vi "Load Configuration.vi"(8 "error in (no error)":errorcluster, 11 "Application in":refnum<class "Application.lvclass">) -> (0 "error out":errorcluster, 3 "Application out":refnum<class "Application.lvclass">)   [LabVIEW 2023, in "Application.lvlib" / "Application.lvclass"]
uses:
  Application.lvclass
  Application.lvclass/Application.ctl
  User Interface/Splash Screen Messages/Update Status Msg/Update Status Msg.lvclass/Update Status Msg.ctl
  <vilib>/ActorFramework/Message Enqueuer/Message Enqueuer.lvclass/Message Enqueuer.ctl
  33bbd52a-dc54-4860-8ff1-e4a75f980f2e.vi
  <vilib>/ActorFramework/Message Enqueuer/Enqueue.vi
  User Interface/Splash Screen Messages/Update Status Msg/Update Status Msg.lvclass
  C:/Program Files/National Instruments/LabVIEW 2023/vi.lib/ActorFramework/Message/Message.lvclass
  <vilib>/ActorFramework/Message Priority Queue/Priority Enqueue.vi
  Resources/GLOBAL/GLOBAL Experiment Metadata.vi
  <vilib>/Utility/xml.llb/Read From XML File(string).vi
  <vilib>/JDP Science/JSONtext/JSON text to Variant.vi
  <vilib>/JDP Science/JSONtext/LVClass Serializer/JSONtext LVClass Serializer.lvclass
panel:
  in  "Edit Button":bool
  in  "Exit":bool
  in  "OK Button":bool
  in  "Select Configuration":u16(ring) items=["Workstation"]
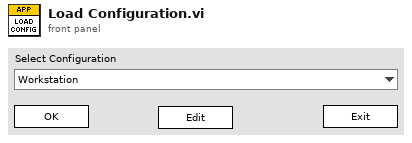
[diagram p1: front panel]
types:
  T1 = cluster{"Hostname":string[], "Config File":string[]}
  T2 = cluster{"filename without extension":string, i32}[]
  T3 = typedef "Hardware Configuration.ctl" = cluster{"Stage Configuration":T4, "Microscope Configuration":T5, "Virtual Camera Configuration":T7, "Laser Configuration":T9[], "Installed Cameras":T10[], "Power Meter Configuration":cluster{"Power Meter Type":enum16{"Disabled", "Thorlabs", "Newport", "Coherent"}, "attenuation":dbl, "instrument handle":refnum<visa-resource-name>}, "DAQ Configuration":T11}
  T4 = typedef "Stage Configuration.ctl" = cluster{"Serial Port":refnum<visa-resource-name>, "Forward Step (mm)":dbl, "Lane Length (mm)":dbl, "Lane Separation (mm)":dbl, "Stage Type":enum16{"Disabled", "ESP301", "Ti2", "Ludl", "ASI", "Simulate"}, "Autofocus Z Planes":i32, "Autofocus Range (um)":dbl, "Stage Limits":cluster{"Y Min":dbl, "Y Max":dbl, "X Min":dbl, "X Max":dbl}, "Slide (mm)":cluster{"top":dbl, "right":dbl, "width":dbl, "height":dbl}}
  T5 = typedef "Microscope Configuration.ctl" = cluster{"Serial Port":refnum<visa-resource-name>, "Microscope Type":T6, "Detection Settings":cluster{"Name":string, "Filter Position":u16, "Optical Path":u16}[]}
  T6 = typedef "Microscope Type.ctl" = enum16{"Disable", "TE2000", "Eclipse Ti", "Ti2"}
  T7 = typedef "Virtual Camera Configuration.ctl" = cluster{"Camera Type":T8}
  T8 = typedef "Camera Type.ctl" = enum16{"Hamamatsu", "Andor", "Photometrics"}
  T9 = typedef "Laser Configuration.ctl" = cluster{"Serial Port":refnum<visa-resource-name>, "Laser Type":enum16{"Disable", "Laser Quantum", "Coherent OBIS", "PRM1-Z8", "Coherent HOPS", "Cobolt"}, "Polarizer Amplitude":dbl, "Polarizer Theta Zero":dbl, "Wavelength":u16}
  T10 = typedef "Physical Camera Assignment.ctl" = cluster{"Channel Name":string, "Serial Number":string, "Flip Vertically":bool, "Flip Horizontally":bool, "wavelength":i16, "photonsPerCount":dbl[]}
  T11 = typedef "DAQ Configuration.ctl" = cluster{"Shutters":T12[], "fluidics trigger line":tag, "camera trigger line":tag, "COM Port":refnum<visa-resource-name>, "Device type":T13}
  T12 = typedef "Shutter Configuration.ctl" = cluster{"IO Line":tag, "Name":string, "Wavelength":u16, "Max rate (Hz)":dbl}
  T13 = typedef "Sync Device Type.ctl" = enum16{"Disabled", "NI DAQ", "Arduino DAQ", "Microsync"}
  T14 = typedef "Default Settings.ctl" = cluster{"Refresh Timeout (ms)":i32, "Version String":string, "Hardware Configuration File":string, "Config Hostname Map":cluster{"Hostname":string[], "Config File":string[]}}
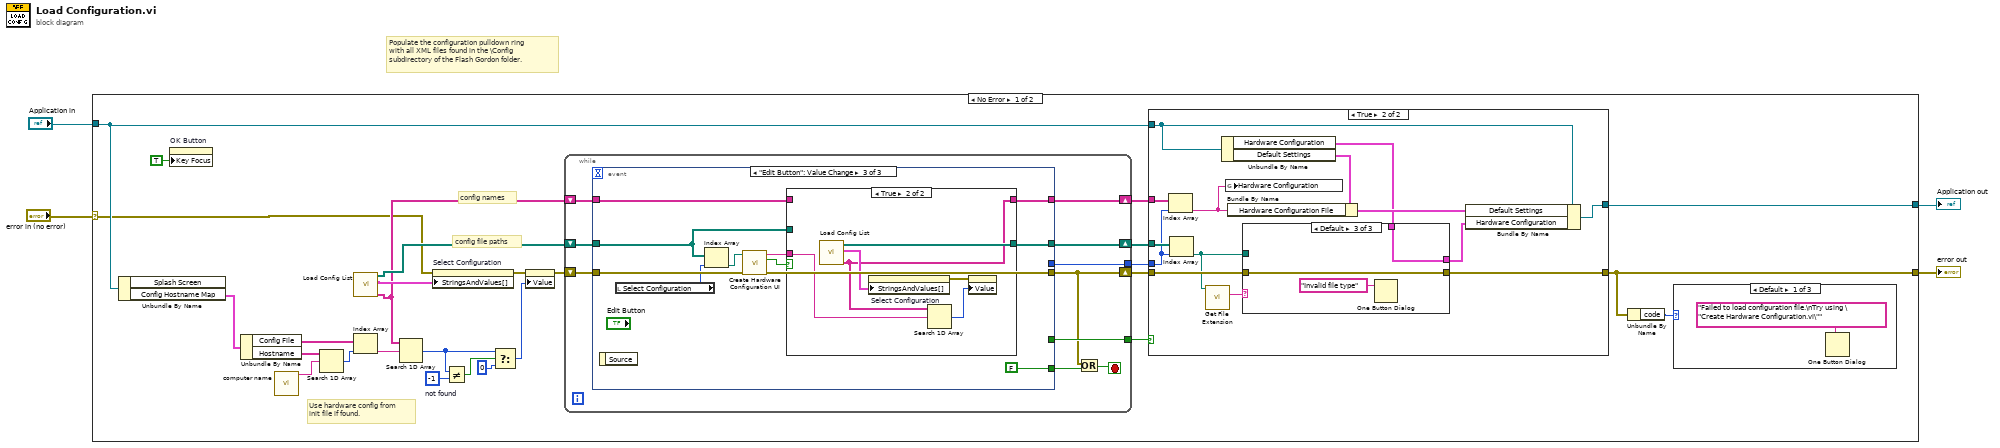
[diagram p0: block diagram]
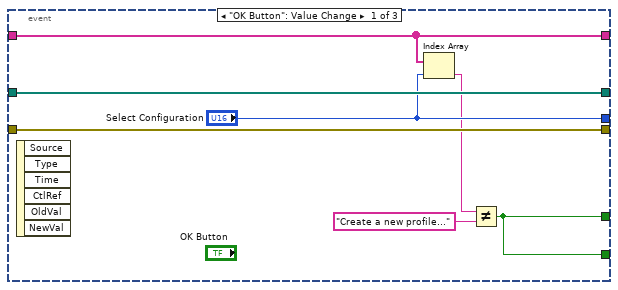
[diagram p2: hidden frame]
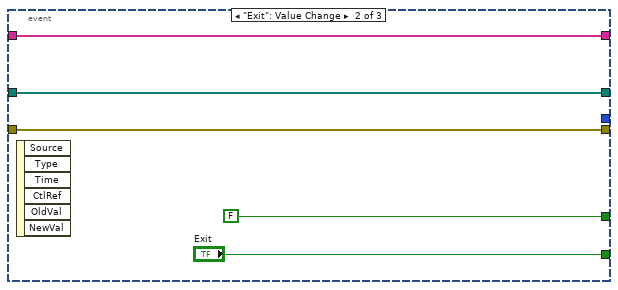
[diagram p3: hidden frame]
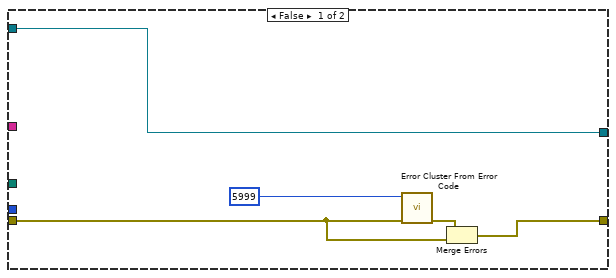
[diagram p5: hidden frame]
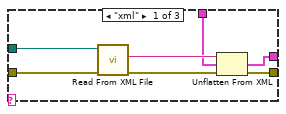
[diagram p6: hidden frame]
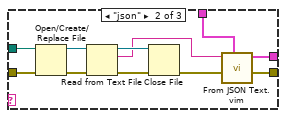
[diagram p7: hidden frame]
diagram:
  # "Populate the configuration pulldown ring\nwith all XML files found in the \\Config\nsubdirectory of the Flash Gordon folder."
  n1 = case shown="No Error" "error in (no error)" {
    selector: "error in (no error)" -> [w5 w115]
    tunnel: [w17 w115] -> w3
    tunnel: [w28 w114] -> w1
    tunnel: "Application in" -> [w16 w114]
    frame No Error {
      w27 = -1  # not found
      # "config file paths"
      # "config names"
      # "Use hardware config from\ninit file if found."
      n2 = Unbundle By Name(w16) -> ("Config Hostname Map"=w15:T1)  [unwired: 1 out]
      n3 = property on="OK Button" class="Bool"("Key Focus"=TRUE) -> ()  [unwired: 2 in, 2 out]
      n4 = Unbundle By Name(w15) -> ("Config File"=w12:string[], "Hostname"=w14:string[])
      n5 = call "computer name.vi"() -> ("name"=w13:string)  [unwired: 11 in]
      n6 = Search 1D Array(1D array=w14, element=w13) -> (index of element=w11:i32)  [unwired: 1 in]
      n7 = call "Load Config List.vi"() -> ("Config Names"=w7:string[], "StringsAndValues[]"=w8:T2, "Config File Paths"=w9:path[])  [unwired: 9 in]
      n8 = Index Array(array=w12, index=w11) -> (element=w10:string)
      n9 = Search 1D Array(1D array=w7, element=w10) -> (index of element=w25:i32)  [unwired: 1 in]
      n10 = property on="Select Configuration" class="Ring (strict)"(error in=w5, "StringsAndValues[]"=w8) -> (error out=w31:errorcluster)  [unwired: 1 in, 1 out]
      n11 = Not Equal?(x=w25, y=w27) -> (x != y?=w26:bool)
      n12 = Select(t=w25, s=w26, f=0) -> (s? t:f=w23:i32)
      n13 = property on="Select Configuration" class="Ring (strict)"(error in=w31, "Value"=w23) -> (error out=w30:errorcluster)  [unwired: 1 in, 1 out]
      n14 = while {
        tunnel: [w36] -> w21
        tunnel: [w35] -> w19
        shift-right: [w32] -> w20
        shift-left: w30 -> [w41]
        shift-right: [w39] -> w29
        shift-left: w9 -> [w40]
        shift-right: [w37] -> w22
        shift-left: w7 -> [w38]
        stop <- w34 stop-if-true
        n15 = event shown="[2] \"Edit Button\": Value Change" {
          selector: _ -> [_ _ _]
          dyn-events: _ -> [_ _ _]
          timeout: _ -> [_ _ _]
          tunnel: w41 -> [w48 w50 w64]
          tunnel: [w48 w50 w63] -> w32
          tunnel: w40 -> [w47 w51 w56]
          tunnel: [w47 w51 w54] -> w39
          tunnel: ["Select Configuration" _ _] -> w36
          tunnel: w38 -> [w45 w52 w57]
          tunnel: [w45 w52 w55] -> w37
          tunnel: [w42 FALSE _] -> w35
          tunnel: [w42 "Exit" FALSE ("Exit")] -> w33
          event "OK Button": Value Change {
            n16 = event-data() -> ()  [unwired: 1 in, 6 out]
            n17 = Index Array(array=w45, index="Select Configuration") -> (element=w44:string)
            n18 = Not Equal?(x=w44, y="Create a new profile...") -> (x != y?=w42:bool)
          }
          event "Exit": Value Change {
            n19 = event-data() -> ()  [unwired: 1 in, 6 out]
          }
          event "Edit Button": Value Change {
            n20 = event-data() -> ()  [unwired: 1 in, 1 out]
            n21 = local read "Select Configuration"() -> (w61:u16)
            n22 = Index Array(array=w56, index=w61) -> (element=w62:path)
            n23 = call "Create Hardware Configuration UI.vi"("error in (no error)"=w64, "Path"=w62) -> ("error out"=w63:errorcluster, "new file?"=w59:bool, "name"=w58:string)  [unwired: 7 in]
            n24 = case shown="True" w59 {
              tunnel: w58 -> [_ w68]
              tunnel: w57 -> [w66 _]
              tunnel: w56 -> [w65 _]
              tunnel: [w66 w69] -> w55
              tunnel: [w65 w72] -> w54
              frame False {
              }
              frame True {
                n25 = call "Load Config List.vi"() -> ("Config Names"=w69:string[], "StringsAndValues[]"=w71:T2, "Config File Paths"=w72:path[])  [unwired: 9 in]
                n26 = property on="Select Configuration" class="Ring (strict)"("StringsAndValues[]"=w71) -> (error out=w70:errorcluster)  [unwired: 2 in, 1 out]
                n27 = Search 1D Array(1D array=w69, element=w68) -> (index of element=w67:i32)  [unwired: 1 in]
                n28 = property on="Select Configuration" class="Ring (strict)"(error in=w70, "Value"=w67) -> ()  [unwired: 1 in, 2 out]
              }
            }
          }
        }
        n29 = Or(x=w32, y=w33) -> (x .or. y?=w34:bool)
      }
      n30 = case shown="True" w19 {
        tunnel: w29 -> [_ w91]
        tunnel: [w77 w90] -> w28
        tunnel: w22 -> [_ w89]
        tunnel: w21 -> [_ w88]
        tunnel: w20 -> [w75 w83]
        tunnel: [w73 w80] -> w17
        tunnel: w16 -> [w77 w85]
        frame False {
          n31 = call <vilib>:"Error Cluster From Error Code.vi"("error in (no error)"=w75, "error code (0)"=5999) -> ("error out"=w76:errorcluster)  [unwired: 7 in]
          n32 = Merge Errors(w76, w75) -> (w73:errorcluster)
        }
        frame True {
          n33 = Index Array(array=w89, index=w88) -> (element=w84:string)
          n34 = Index Array(array=w91, index=w88) -> (element=w78:path)
          n35 = call <vilib>:"Get File Extension.vi"("file"=w78) -> ("lowercase file extension"=w79:string)  [unwired: 6 in, 4 out]
          n36 = Unbundle By Name(w85) -> ("Hardware Configuration"=w82:T3, "Default Settings"=w87:T14)
          n37 = global write "GLOBAL Experiment Metadata.vi" "Hardware Configuration"(w84) -> ()
          n38 = Bundle By Name(cluster=w87, "Hardware Configuration File"=w84) -> (w86:T14)
          n39 = case shown="Default" w79 {
            tunnel: w83 -> [w97 w109 w111]
            tunnel: w78 -> [w98 w108 _]
            tunnel: w82 -> [w92 w101 w112]
            tunnel: [w94 w100 w112] -> w81
            tunnel: [w95 w99 w111] -> w80
            frame "xml" {
              n40 = call-poly <vilib>:"Read From XML File.vi"("error in (no error)"=w97, "XML File Path"=w98) -> ("error out"=w96:errorcluster, "XML Elements"=w93:string)  [unwired: 7 in, 1 out]
              n41 = Unflatten From XML(xml string=w93, type=w92, error in (no error)=w96) -> (value=w94:T3, error out=w95:errorcluster)
            }
            frame "json" {
              n42 = Open/Create/Replace File(file path (use dialog)=w108, error in=w109) -> (refnum out=w106:refnum<file>, error out=w107:errorcluster)  [unwired: 4 in, 1 out]
              n43 = Read from Text File(file (use dialog)=w106, error in=w107) -> (refnum out=w105:refnum<file>, text=w103:string, error out=w104:errorcluster)  [unwired: 2 in, 1 out]
              n44 = Close File(refnum=w105, error in=w104) -> (error out=w102:errorcluster)  [unwired: 1 out]
              n45 = call "From JSON Text.vim"("Data Type and Default Value"=w101, "error in (no error)"=w102, "JSON"=w103) -> ("error out"=w99:errorcluster, "Data out"=w100:T3)  [unwired: 7 in]
            }
            frame Default {
              n46 = One Button Dialog(message="Invalid file type") -> ()  [unwired: 1 in, 1 out]
            }
          }
          n47 = Bundle By Name(cluster=w85, "Default Settings"=w86, "Hardware Configuration"=w81) -> (w90:refnum<class "Application.lvclass">)
        }
      }
      n48 = Unbundle By Name(w17) -> ("code"=w18:i32)
      n49 = case shown="Default" w18 {
        frame Default {
          n50 = One Button Dialog(message="Failed to load configuration file.\nTry using \"Create Hardware Configuration.vi\"") -> ()  [unwired: 1 in, 1 out]
        }
        frame 0 {
          # "no error"
        }
        frame 5999 {
          # "User hit \"Cancel\" in dialog to load a configuration"
        }
      }
    }
    frame Error {
    }
  }
  "error out" <- w3
  "Application out" <- w1
